vi "HW Configure.vi"(6 "Acquired z-plane index":i32, 8 "Error In":errorcluster) -> (0 "Error Out":errorcluster, 3 "AOL_Globals":T1={"Imaging Protocol"=enum."Live Imaging", "Number of POI"=0, "Number of Miniscans"=0, "Number of Trials"=0, "Number of Cycles "=0, "# Averaged Frames"=0, "Laser power (%)"=0, "Pockels (V)"=0.0, "Acquisition Length (sec)"=0.0, "Fill time (us)"=0.0, "POI Dwell time (us)"=0.0, "Miniscan Dwell time per pixel (us)"=0.0, "PMT 1"=0.0, "PMT 2"=0.0, "Back Apperture (mA)"=0.0, "Frame Size"=200, "Center Frequency"=0.0, "Field of View (um)"=175.0, "Field of View (norm)"=0.0, "DwellTime (us)"=0.0, "Ref Dwell Time (us)"=0.0, "Wavelength (nm)"=0.0, "Zoom"=0.0, "AOL Z"=0.0, "AOL Mode"=enum."Raster", "GridXY"=0.0, "GridZ"=0.0, "TriggerPeriod (sec)"=0.0, "Number of Pixels in Miniscan"=0, "Experiment folder path"=path "", "X centre"=0.0, "Y centre"=0.0, "Angle (degrees)"=0.0, "Angle Xs (degrees)"=0.0, "Angle Ys (degrees)"=0.0, "Plane Mode"=0, "Threshold"=[], "Regenerate Chirps"=FALSE, "Rectangle ROI length (pixels)"=0, "Rectangle ROI height (pixels)"=0, "AOD fill"=4900, "StartupDelay"=0, "Samples Wait after Trigger"=5080, "Slip Cycle"=600000, "Add Cycle"=TRUE, "Functional Mode"=enum."Point", "Z Start"=0.0, "Z Stop"=0.0, "# Planes"=0, "Total Pixels"=0, "Variable Miniscan Pixels"=[], "Use Variable Length"=FALSE, "Use Variable Resolution"=FALSE, "Laser power (%) at Z Start"=0, "Laser power (%) at Z Stop"=0, "Ref Z Step"=0} {"Angle Ys (degrees)" format="%#.6g"; "Angle Xs (degrees)" format="%#.6g"; "Plane Mode" items=["XY Plane", "XZ Plane", "YZ Plane", "arbitraryplane"]; "Frame Size" items=["100X100"=100, "128X128"=128, "200X200"=200, "256X256"=256, "512X512"=512, "1024x1024"=1024, "2048x2048"=2048]; "Back Apperture (mA)" format="%#.6g"; "Pockels (V)" format="%#.6g"; "PMT 2" format="%#.6g"; "PMT 1" format="%#.6g"; "Angle (degrees)" format="%#.6g"; "POI Dwell time (us)" format="%#.6g"})   [LabVIEW 2020]
doc: "Configure the hardware."
uses:
  Typedefs/Controls/AOL_Globals.ctl
  Typedefs/Imaging Protocols enum.ctl
  Typedefs/Frame Size.ctl
  Typedefs/AOL modes.ctl
  Typedefs/Plane Mode.ctl
  Typedefs/Functional Mode.ctl
  Typedefs/Shutter Function Enum.ctl
panel:
  out "Execution time":u32
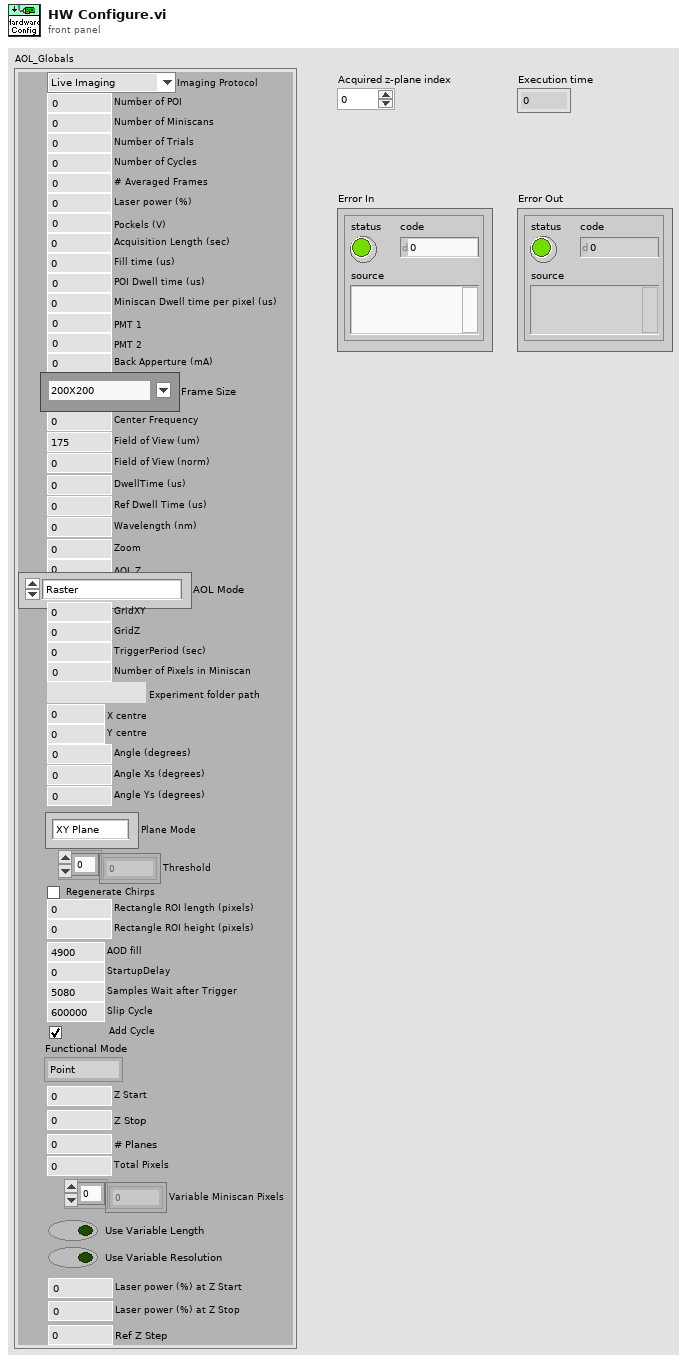
[diagram p1: front panel]
types:
  T1 = typedef "AOL_Globals.ctl" = cluster{"Imaging Protocol":T2, "Number of POI":u16, "Number of Miniscans":u16, "Number of Trials":u16, "Number of Cycles ":u64, "# Averaged Frames":u16, "Laser power (%)":u8, "Pockels (V)":dbl, "Acquisition Length (sec)":dbl, "Fill time (us)":dbl, "POI Dwell time (us)":dbl, "Miniscan Dwell time per pixel (us)":dbl, "PMT 1":dbl, "PMT 2":dbl, "Back Apperture (mA)":dbl, "Frame Size":T3, "Center Frequency":dbl, "Field of View (um)":dbl, "Field of View (norm)":dbl, "DwellTime (us)":dbl, "Ref Dwell Time (us)":dbl, "Wavelength (nm)":dbl, "Zoom":dbl, "AOL Z":dbl, "AOL Mode":T4, "GridXY":dbl, "GridZ":dbl, "TriggerPeriod (sec)":dbl, "Number of Pixels in Miniscan":u16, "Experiment folder path":path, "X centre":dbl, "Y centre":dbl, "Angle (degrees)":dbl, "Angle Xs (degrees)":dbl, "Angle Ys (degrees)":dbl, "Plane Mode":T5, "Threshold":u16[], "Regenerate Chirps":bool, "Rectangle ROI length (pixels)":u16, "Rectangle ROI height (pixels)":u16, "AOD fill":u16, "StartupDelay":i32, "Samples Wait after Trigger":u16, "Slip Cycle":u32, "Add Cycle":bool, "Functional Mode":T6, "Z Start":dbl, "Z Stop":dbl, "# Planes":i32, "Total Pixels":i32, "Variable Miniscan Pixels":u16[], "Use Variable Length":bool, "Use Variable Resolution":bool, "Laser power (%) at Z Start":u8, "Laser power (%) at Z Stop":u8, "Ref Z Step":i8}
  T2 = typedef "Imaging Protocols enum.ctl" = enum16{"AOL Z-Stack", "Motor Z Stack", "Parameter Sweep", "Functional Acquisition", "Single Plane Acquisition", "Volume Acquisition", "Live Imaging", "Live Plane Imaging", "Live Volume Imaging"}
  T3 = typedef "Frame Size.ctl" = u16
  T4 = typedef "AOL modes.ctl" = enum16{"Raster", "Structural", "Pointing", "Mini Scan", "Alignment"}
  T5 = typedef "Plane Mode.ctl" = u16
  T6 = typedef "Functional Mode.ctl" = enum16{"Point", "Line", "Patch", "Plane", "Volume"}
  T7 = typedef "Shutter Function Enum.ctl" = enum16{"Open Shutter", "Close Shutter"}
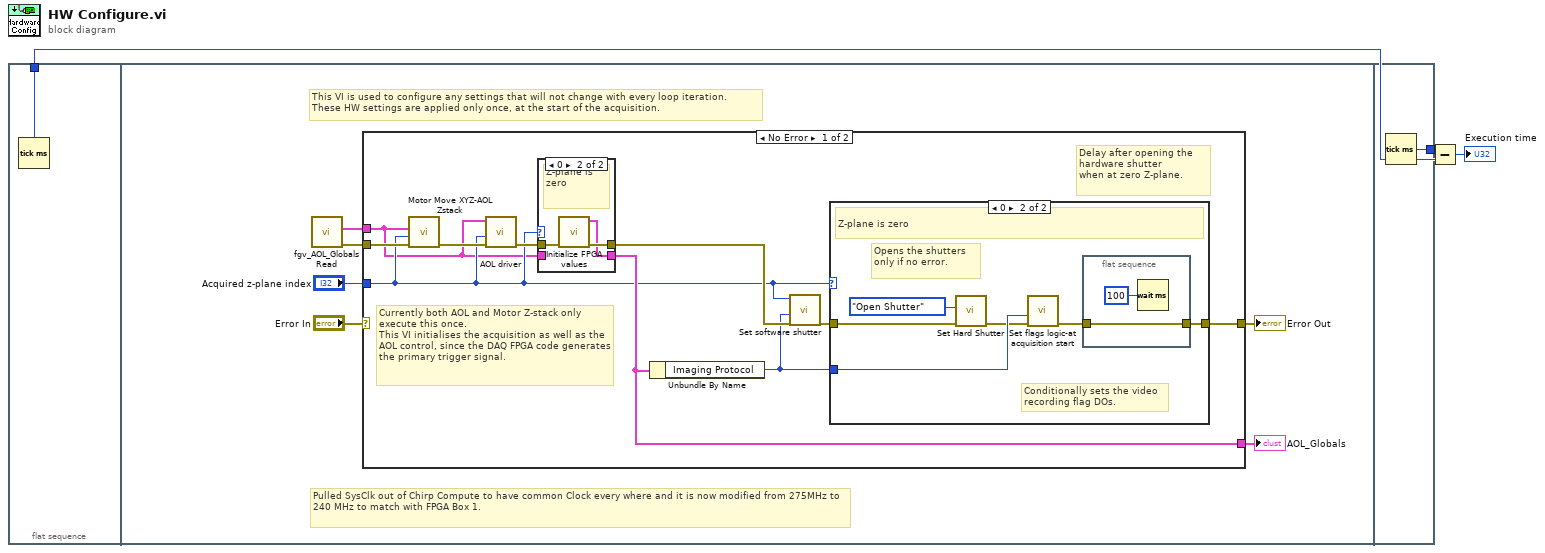
[diagram p0: block diagram]
diagram:
  n1 = flat-sequence {
    tunnel: [w4] -> w2
    tunnel: [w36] -> w3
    frame #0 {
      n2 = Tick Count (ms)() -> (millisecond timer value=w4:u32)
    }
    frame #1 {
      # "Pulled SysClk out of Chirp Compute to have common Clock every where and it is now modified from 275MHz to 240 MHz to match with FPGA Box 1."
      # "This VI is used to configure any settings that will not change with every loop iteration.\nThese HW settings are applied only once, at the start of the acquisition."
      n3 = call "fgv_AOL_Globals Read.vi"() -> ("error out"=w5:errorcluster, "AOL_Globals"=w6:T1)  [unwired: 9 in, 1 out]
      n4 = case shown="No Error" "Error In" {
        selector: "Error In" -> [_ w35]
        tunnel: [w20 w35] -> w9
        tunnel: "Acquired z-plane index" -> [w12 _]
        tunnel: [w14 _] -> w7
        tunnel: w6 -> [w11 _]
        tunnel: w5 -> [w19 _]
        frame No Error {
          # "Delay after opening the hardware shutter\nwhen at zero Z-plane."
          # "Currently both AOL and Motor Z-stack only execute this once.\nThis VI initialises the acquisition as well as the AOL control, since the DAQ FPGA code generates the primary trigger signal."
          n5 = call "Motor Move XYZ-AOL Zstack.vi"("error in (no error)"=w19, "Zplane in"=w12, "AOL_Globals"=w11) -> ("error out"=w13:errorcluster)  [unwired: 8 in]
          n6 = call "AOL driver.vi"("Error in"=w13, "Acquired z-plane index / volume index"=w12, "AOL_Globals"=w11) -> ("Error out"=w18:errorcluster)  [unwired: 8 in]
          n7 = case shown="0" w12 {
            tunnel: [w31 w34] -> w17
            tunnel: w18 -> [w31 w33]
            tunnel: w11 -> [w30 _]
            tunnel: [w30 w32] -> w14
            frame Default {
              # "Consecutive plane to be acquired"
            }
            frame 0 {
              # "Z-plane is zero"
              n8 = call "Initialize FPGA values.vi"("Error In"=w33) -> ("Error Out"=w34:errorcluster, "AOL_Globals"=w32:T1)  [unwired: 9 in]
            }
          }
          n9 = Unbundle By Name(w14) -> ("Imaging Protocol"=w15:T2)
          n10 = call "Set software shutter.vi"("error in (no error)"=w17, "Imaging Protocol"=w15, "Acquired z-plane index"=w12) -> ("Error Out"=w16:errorcluster)  [unwired: 8 in]
          n11 = case shown="0" w12 {
            tunnel: [w21 w22] -> w20
            tunnel: w16 -> [w21 w26]
            tunnel: w15 -> [_ w25]
            frame Default {
              # "Any z-plane other than zero"
            }
            frame 0 {
              # "Conditionally sets the video recording flag DOs."
              # "Opens the shutters only if no error."
              # "Z-plane is zero"
              n12 = call "Set Hard Shutter.vi"("Error In"=w26, "Shutter Function"=Shutter_Function_Enum."Open Shutter") -> ("Error Out"=w23:errorcluster)  [unwired: 9 in]
              n13 = call "Set flags logic-at acquisition start.vi"("error in (no error)"=w23, "Imaging Protocol"=w25) -> ("error out"=w24:errorcluster)  [unwired: 9 in]
              n14 = flat-sequence {
                tunnel: w24 -> [w29]
                tunnel: [w29] -> w22
                frame #0 {
                  n15 = Wait (ms)(milliseconds to wait=u32 100) -> ()  [unwired: 1 out]
                }
              }
            }
          }
        }
        frame Error {
        }
      }
      "Error Out" <- w9
      "AOL_Globals" <- w7
    }
    frame #2 {
      n16 = Tick Count (ms)() -> (millisecond timer value=w36:u32)
    }
  }
  n17 = Subtract(x=w3, y=w2) -> (x-y=→"Execution time":u32)
